vi "ADC SNR_Sweep_edited.vi"(8 "error in (no error)":errorcluster, 9 "Sequence parameters":string[][](array[string])=[["Min limit", "Max limit", "Register sheet file", "Register Sheet"], ["", "", "CC2600.xls", "TX_BLE;Trim"], ["Reg write (addr;value)", "Operating frequency [Hz]", "", ""], ["NA", "2.44G", "", ""]], 10 "Run type":i32, 11 "Method parameters":T3={"Dev"={"Do not disturb DUT"=FALSE, "XOSC"=32000000.0, "Board type"="", "EM"="", "Configure tempboard"=TRUE, "Device specific info"=[], "Generic Object"=refnum}, "Method"={"Run type"=1, "Test name"="Current LPM2 4", "Comment"="", "Results folder"="", "AFC"=enum."Off", "Method name"="Current LPM2 4", "Method results"={"Excel brief report"=FALSE, "Spotfire report"=FALSE, "Starfish report"=FALSE}, "Operator"="", "Reference time"=timestamp(0 s since 1904-01-01), "AFC delay"=0.0, "Initialization"=enum."Enabled", "MD5 Sum"="", "HW addon board"=enum."None", "AFC Regsheet"="", "AFC Regfile"=path "", "dummy"=0.0}, "Inst"={"Instr"={"PS1"={"Name"="", "GPIB address"="", "VISA session"=""}, "PS2"={"Name"="", "GPIB address"="", "VISA session"=""}, "TC1"={"Name"="", "GPIB address"="", "VISA session"=""}, "TC2"={"Name"="", "GPIB address"="", "VISA session"=""}, "SA1"={"Name"="", "GPIB address"="", "VISA session"=""}, "SA2"={"Name"="", "GPIB address"="", "VISA session"=""}, "SG1"={"Name"="", "GPIB address"="", "VISA session"=""}, "SG2"={"Name"="", "GPIB address"="", "VISA session"=""}, "SG3"={"Name"="", "GPIB address"="", "VISA session"=""}, "MI1"={"Name"="", "GPIB address"="", "VISA session"=""}, "MI2"={"Name"="", "GPIB address"="", "VISA session"=""}, "SW SA"={"Name"="", "Controller addr"=""}, "SW SG"={"Name"="", "Controller addr"=""}, "MI3"={"Name"="", "GPIB address"="", "VISA session"=""}}, "Switchbox"={"RF Path"=0, "Cal compensation"=enum."TX", "Switchbox gain mode"="", "State"=enum."TX"}, "Instr to control (i.e. SA1)"="Default", "Intrument info string"=""}, "Sequence parameters"=[["Weight", "Min Limit", "Max Limit", "Register Sheet", "", "", "", "", "", "", "", "", ""], ["Vital", "", "1", "LPM2", "", "", "", "", "", "", "", "", ""], ["Resolution", "Reg write (addr;value)", "Chip mode", "Range", "", "", "", "", "", "", "", "", ""], ["u", "NA", "", "auto", "", "", "", "", "", "", "", "", ""]], "Cond"={"Temp logged"=25.0, "VDD1_PS1_6V"=-999.0, "VDD2_PS1_25V"=-999.0, "VDD4_PS2_25V"=-999.0, "VDD3_PS2_6V"=-999.0}, "Meas config"={"X-axis inner loop index"=32000000, "Y-axis outer loop index"=32000000, "X-axis"=[], "Y-axis"=[], "X-axis array req size"=32000000, "Y-axis array req size"=32000000, "Param description"=[], "Use meas clust for reporting"=FALSE, "Parameter index (page)"=0, "X-axis name"="", "Y-axis name"=""}} {"Cond"."VDD3_PS2_6V" format="%.3f"; "Cond"."VDD4_PS2_25V" format="%.3f"; "Cond"."VDD2_PS1_25V" format="%.3f"; "Cond"."VDD1_PS1_6V" format="%.3f"; "Method"."dummy" format="%.1p"; "Method"."AFC delay" format="%.1p"; "Dev"."XOSC" format="%.3p"}) -> (0 "error out":errorcluster, 1 "End method error":T1, 2 "Short Results":string[](array[string]), 3 "Result summary":string[][](array[string])=[["Critical", "Output Power@2405 MHz", "-3", "4", "dBm"], ["Critical", "Output Power@2410 MHz", "-3", "4", "dBm"]])   [LabVIEW 2019]
doc: "[AutoDocStart]Performs crystal accuracy measurements. Measures the offset from ideal frequency. Primarily used for tuning XOSC capacitors and verifying XOSC trims.\n\nSweeping parameters: operating frequency, OSC override value and VDDR level\n\nResults: Offset frequency in ppm[AutoDocEnd]"
uses:
  User Lib/Utilities/Cluster definitions/Method input.ctl
  User Lib/Utilities/Cluster definitions/Device specific info.ctl
  User Lib/Utilities/Controls/Automatic Frequency Compensation types.ctl
  User Lib/Utilities/Controls/Method Reports.ctl
  User Lib/Utilities/Cluster definitions/Method Initialization.ctl
  User Lib/Utilities/Controls/HW addon boards.ctl
  User Lib/Utilities/Cluster definitions/Instr clust.ctl
  User Lib/Utilities/Switchbox control/SwitchBox_State._ENUMctl.ctl
  User Lib/Utilities/Cluster definitions/End method error cluster.ctl
  d1e189ac-5c6c-49e1-a56b-a93f7ba1e5c3.vi
  89ac9e08-f822-48c3-bf7b-b9620a48f2c1.vi
  afbe0b8a-4628-4f4a-a689-fb3560c1b1a6.vi
  160c279e-5860-4c4e-a522-43dd8a66307b.vi
  eb3a7dab-0138-448e-bc0a-4bb49588a4f1.vi
  4ae92598-944e-459b-8fa7-3a23a971f601.vi
  e1f832d6-75bf-4ba2-931c-48c142ce58ac.vi
panel:
  in  "Tab Control":T2(tab)
  # "°C"
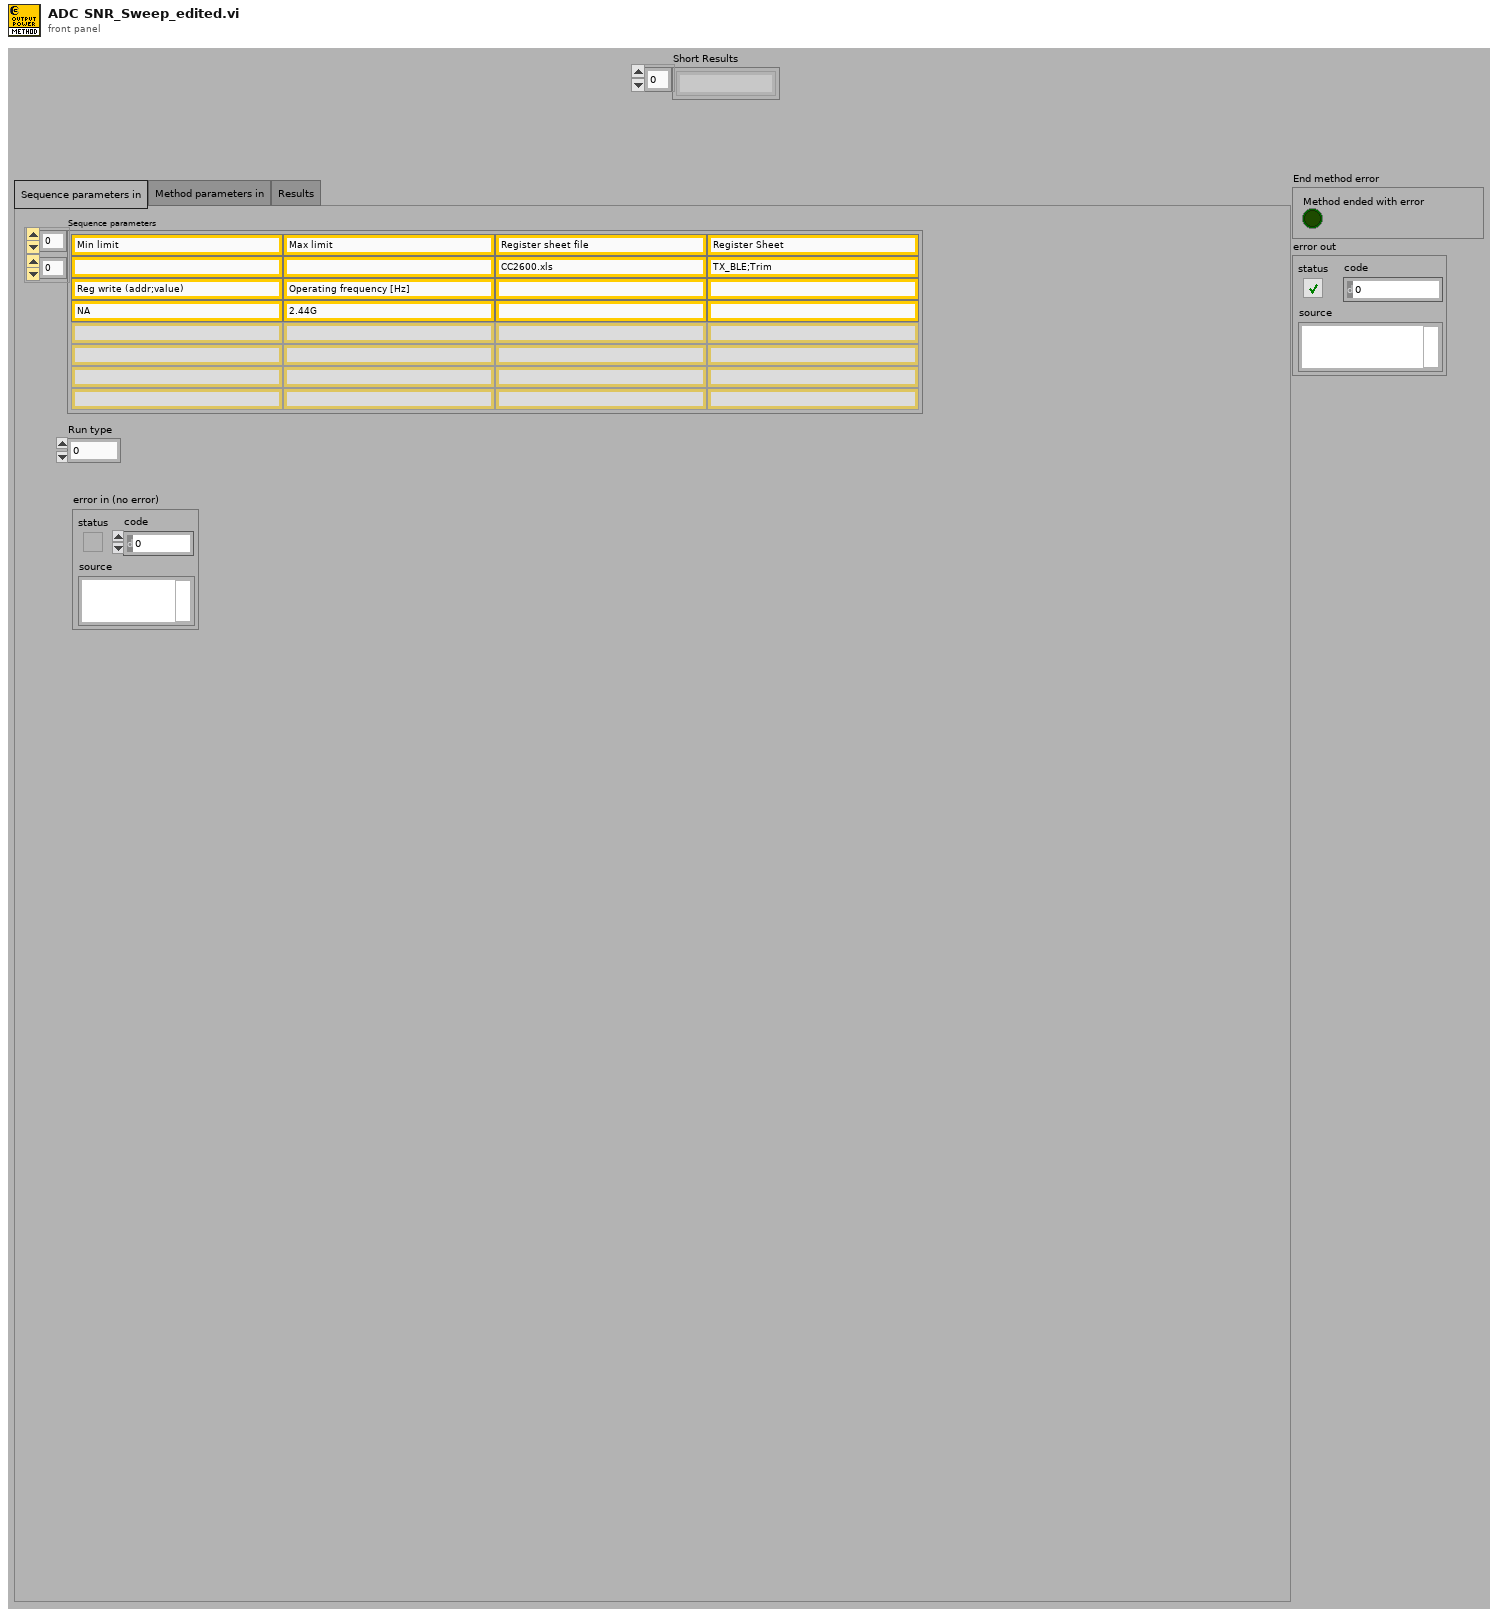
[diagram p1: front panel]
types:
  T1 = typedef "End method error cluster.ctl" = cluster{"Method ended with error":bool}
  T2 = enum32{"Sequence parameters in", "Method parameters in", "Results"}
  T3 = typedef "Method input.ctl" = cluster{"Dev":cluster{"Do not disturb DUT":bool, "XOSC":dbl, "Board type":string, "EM":string, "Configure tempboard":bool, "Device specific info":T4[], "Generic Object":refnum<class>}, "Method":cluster{"Run type":i32, "Test name":string, "Comment":string, "Results folder":string, "AFC":T5, "Method name":string, "Method results":T6, "Operator":string, "Reference time":timestamp, "AFC delay":dbl, "Initialization":T7, "MD5 Sum":string, "HW addon board":T8, "AFC Regsheet":string, "AFC Regfile":path, "dummy":dbl}, "Inst":T9, "Sequence parameters":string[][], "Cond":cluster{"Temp logged":dbl, "VDD1_PS1_6V":dbl, "VDD2_PS1_25V":dbl, "VDD4_PS2_25V":dbl, "VDD3_PS2_6V":dbl}, "Meas config":cluster{"X-axis inner loop index":i32, "Y-axis outer loop index":i32, "X-axis":string[], "Y-axis":string[], "X-axis array req size":i32, "Y-axis array req size":i32, "Param description":string[][], "Use meas clust for reporting":bool, "Parameter index (page)":i32, "X-axis name":string, "Y-axis name":string}}
  T4 = typedef "Device specific info.ctl" = cluster{"EM number":u8, "IP address":string, "Enabled":bool, "Slot no":u8, "RF path":u8, "EM name":string, "Wafer info":string, "AFC frequency ppm":dbl, "Register writes":string[][], "Meas data":string[][][], "Device comment":string}
  T5 = typedef "Automatic Frequency Compensation types.ctl" = enum16{"Off", "Compensate Instrument frequency", "Compensate DUT frequency", "Predictive - Compensate Instrument frequency", "Predictive - Compensate DUT frequency", "Do not skip re-init - Compensate Instrument frequency", "Do not skip re-init - Compensate DUT frequency"}
  T6 = typedef "Method Reports.ctl" = cluster{"Excel brief report":bool, "Spotfire report":bool, "Starfish report":bool}
  T7 = typedef "Method Initialization.ctl" = enum16{"Enabled", "Skip Instr and Device Init", "Enabled with Separate Flash", "Set PS, Device Init and Skip Instr Init", "Skip Device Init"}
  T8 = typedef "HW addon boards.ctl" = enum16{"None", "Current meas 5EM", "Stresstest 10EM"}
  T9 = typedef "Instr clust.ctl" = cluster{"Instr":cluster{"PS1":cluster{"Name":string, "GPIB address":string, "VISA session":refnum<visa-resource-name>}, "PS2":cluster{"Name":string, "GPIB address":string, "VISA session":refnum<visa-resource-name>}, "TC1":cluster{"Name":string, "GPIB address":string, "VISA session":refnum<visa-resource-name>}, "TC2":cluster{"Name":string, "GPIB address":string, "VISA session":refnum<visa-resource-name>}, "SA1":cluster{"Name":string, "GPIB address":string, "VISA session":refnum<visa-resource-name>}, "SA2":cluster{"Name":string, "GPIB address":string, "VISA session":refnum<visa-resource-name>}, "SG1":cluster{"Name":string, "GPIB address":string, "VISA session":refnum<visa-resource-name>}, "SG2":cluster{"Name":string, "GPIB address":string, "VISA session":refnum<visa-resource-name>}, "SG3":cluster{"Name":string, "GPIB address":string, "VISA session":refnum<visa-resource-name>}, "MI1":cluster{"Name":string, "GPIB address":string, "VISA session":refnum<visa-resource-name>}, "MI2":cluster{"Name":string, "GPIB address":string, "VISA session":refnum<visa-resource-name>}, "SW SA":cluster{"Name":string, "Controller addr":string}, "SW SG":cluster{"Name":string, "Controller addr":string}, "MI3":cluster{"Name":string, "GPIB address":string, "VISA session":refnum<visa-resource-name>}}, "Switchbox":cluster{"RF Path":i32, "Cal compensation":enum16{"TX", "RX", "Interferer", "No compensation", "Interferer2"}, "Switchbox gain mode":string, "State":T10}, "Instr to control (i.e. SA1)":string, "Intrument info string":string}
  T10 = typedef "SwitchBox_State._ENUMctl.ctl" = enum16{"TX", "RX", "SP:TX", "SP:RX", "SW:TX", "SW:RX"}
  T11 = cluster{"Fundamental Frequency":dbl, "Sampling Frequncy":dbl, "No of Harmonics":u8, "Window":enum16{"None ", "Hanning", "Hamming", "Blackman-Harris", "Exact Blackman", "Blackman", "Flat Top", "4 Term B-Harris ", "7 Term B-Harris"}, "Blackman (fundamental power) bins)":dbl}
  T12 = enum32{"NI Card Settings", "Memory Read Setting", "DC Capture", "ADC Ramp", "ADC Sine", "SNR", "Cap Calibration"}
  T13 = enum32{"Read from Memory", "Read .dat file", "NI Card Capture", "None"}
  T14 = cluster{"Path to Save plot":path, "Path to Raw Data plot":path}
  T15 = cluster{"Save INL/DNL Plot(Ramp)":bool, "Save SNR Plot":bool, "Save INL/DNL Plot(Sine)":bool, "Save INL/DNL Raw Data(Ramp)":bool, "Save SNR Raw Data":bool, "Save INL/DNL Raw Data(Sine)":bool, "Save DC Raw data":bool, "Save  Raw Data(Sine)":bool}
  T16 = cluster{"SNR":dbl, "SNRD":dbl, "THD":dbl, "ENOB (SNRD)":dbl, "SFDR":dbl, "ENOB (SNR)":dbl, "Noise Power":dbl, "Signal power":dbl}
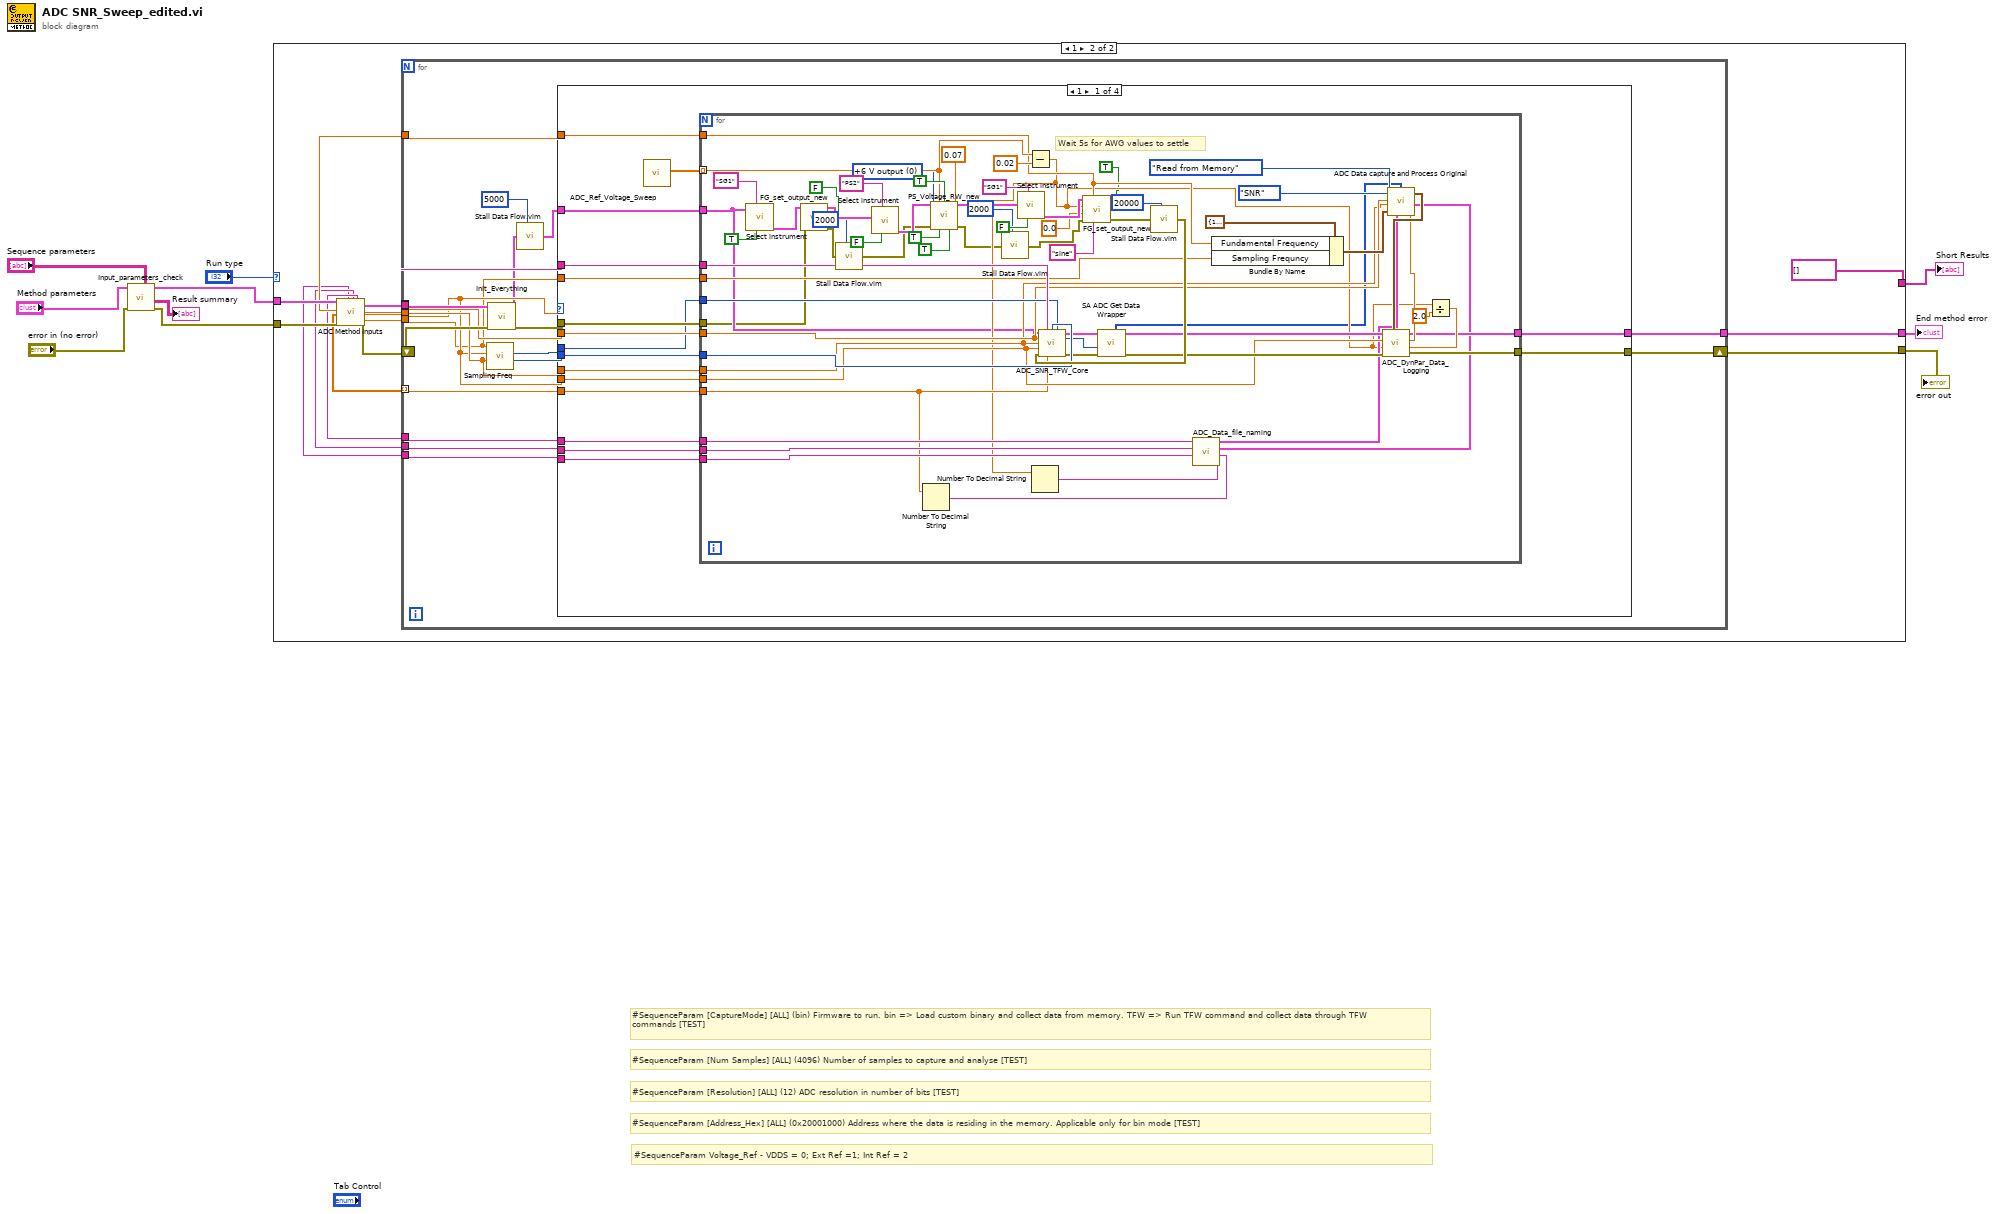
[diagram p0: block diagram]
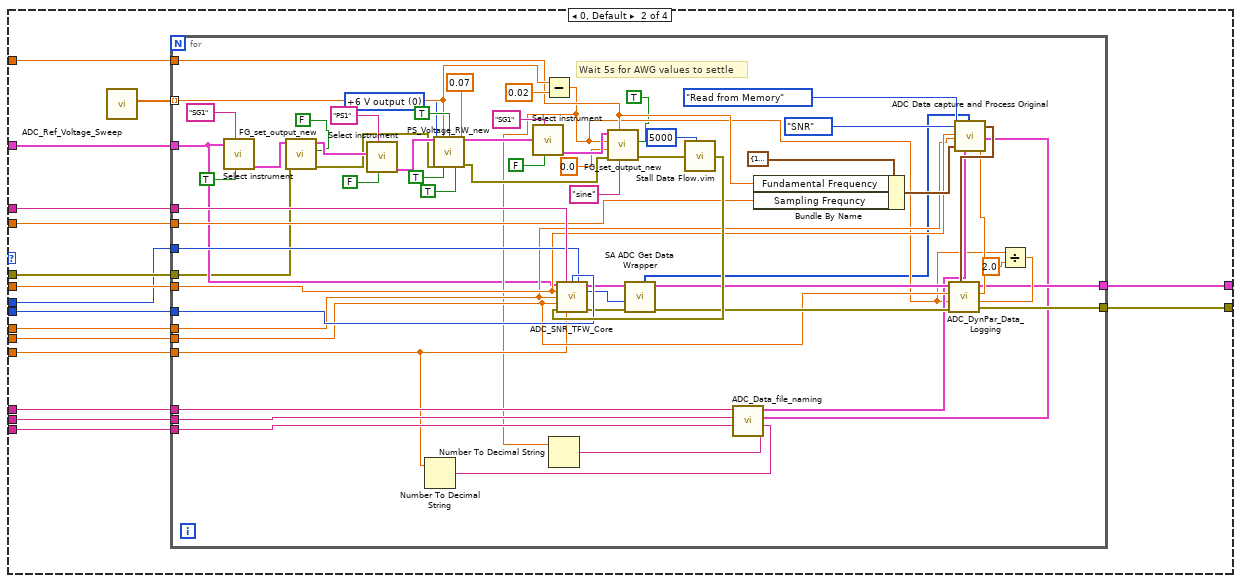
[diagram p3: hidden frame]
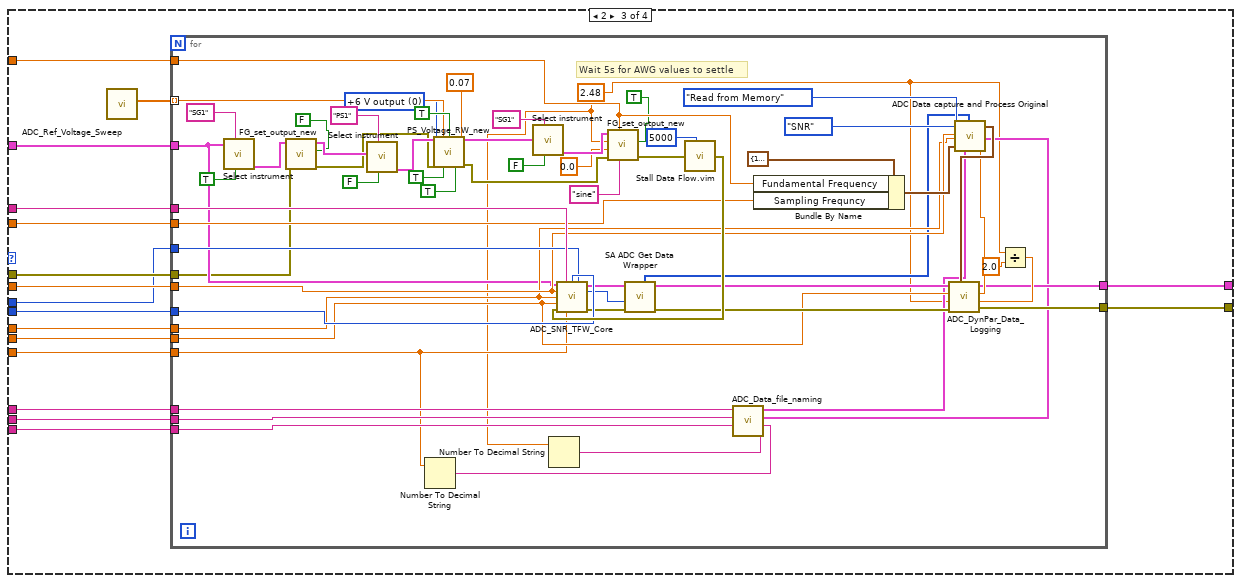
[diagram p4: hidden frame]
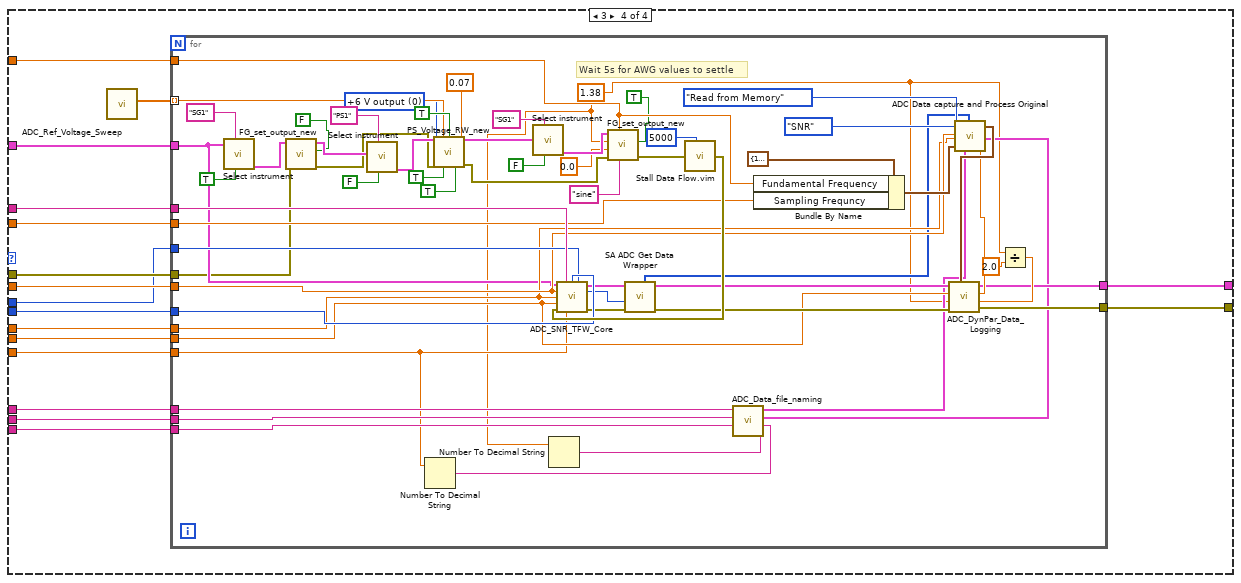
[diagram p5: hidden frame]
diagram:
  # "#SequenceParam Voltage_Ref - VDDS = 0; Ext Ref =1; Int Ref = 2"
  # "#SequenceParam [Num Samples] [ALL] (4096) Number of samples to capture and analyse [TEST]"
  # "#SequenceParam [CaptureMode] [ALL] (bin) Firmware to run. bin => Load custom binary and collect data from memory. TFW => Run TFW command and collect data through TFW commands [TEST]"
  # "#SequenceParam [Address_Hex] [ALL] (0x20001000) Address where the data is residing in the memory. Applicable only for bin mode [TEST]"
  # "#SequenceParam [Resolution] [ALL] (12) ADC resolution in number of bits [TEST]"
  n1 = call "Input_parameters_check.vi"("Sequence parameters"="Sequence parameters", "error in"="error in (no error)", "Method cluster in"="Method parameters") -> ("error out"=w10:errorcluster, "Result summary"=→"Result summary":string[][], "Method cluster out"=w6:T3)  [unwired: 6 in]
  n2 = case shown="1" "Run type" {
    tunnel: w10 -> [w11 w28]
    tunnel: w6 -> [_ w27]
    tunnel: [string[] [] string[] []] -> w3
    tunnel: [w11 w18] -> w2
    tunnel: [_ w17] -> w1
    frame 0, Default {
      # "Run type 0 is only for formatting the result summary"
    }
    frame 1 {
      n3 = call "ADC Method Inputs.vi"("Method cluster in"=w27, "error in (no error)"=w28) -> ("Capture Mode"=w21:string, "Signal Freq"=w20:dbl, "ADC Chnl No."=w13:dbl[], "Sampling Freq String"=w14:string, "Resolution String"=w15:string, "Voltage Ref String"=w16:string, "Method cluster out"=w26:T3, "Num Samples"=w24:dbl, "Resolution"=w23:dbl, "Voltage Ref"=w22:dbl, "Sampling Freq"=w19:dbl, "error out"=w25:errorcluster)  [unwired: 6 in]
      n4 = for {
        tunnel: w26 -> [w49]
        tunnel: w24 -> [w46]
        tunnel: w23 -> [w45]
        tunnel: w22 -> [w44]
        tunnel: w21 -> [w43]
        tunnel: w20 -> [w40]
        tunnel: w19 -> [w39]
        tunnel: [w37] -> w17
        tunnel: w16 -> [w36]
        tunnel: w15 -> [w35]
        tunnel: w14 -> [w34]
        shift-right: [w38] -> w18
        shift-left: w25 -> [w48]
        tunnel: w13 -> [w33] mode=indexing
        n5 = call "Sampling Freq.vi"("Resolution"=w45, "Voltage Ref"=w44, "Sampling Freq"=w39) -> ("LGPT Count"=w42:u16, "SCOMP"=w41:u16)  [unwired: 7 in]
        n6 = call "Init_Everything.vi"("error in"=w48, "Method cluster In"=w49) -> ("error out"=w47:errorcluster, "Method cluster out"=w31:T3)  [unwired: 6 in, 2 out]
        n7 = call "Stall Data Flow.vim"("value in"=w31, "milliseconds to wait"=u32 5000) -> ("value out"=w32:T3)  [unwired: 1 out]
        n8 = case shown="1" w44 {
          tunnel: w32 -> [w65 w148 w227 w305]
          tunnel: w47 -> [w64 w147 w226 w304]
          tunnel: w46 -> [w63 w146 w225 w303]
          tunnel: w45 -> [w62 w145 w224 w302]
          tunnel: w44 -> [w61 w144 w223 w301]
          tunnel: w43 -> [w60 w143 w222 w300]
          tunnel: w42 -> [w59 w142 w221 w299]
          tunnel: w41 -> [w58 w141 w220 w298]
          tunnel: w40 -> [w57 w140 w219 w297]
          tunnel: w33 -> [w56 w139 w218 w296]
          tunnel: w39 -> [w55 w138 w217 w295]
          tunnel: [w54 w137 w216 w294] -> w37
          tunnel: [w53 w136 w215 w293] -> w38
          tunnel: w36 -> [w52 w135 w214 w292]
          tunnel: w35 -> [w51 w134 w213 w291]
          tunnel: w34 -> [w50 w133 w212 w290]
          frame 1 {
            n9 = call "ADC_Ref_Voltage_Sweep.vi"() -> ("Ref voltage sweep"=w66:dbl[])  [unwired: 11 in]
            n10 = for {
              tunnel: w66 -> [w112] mode=indexing
              tunnel: w65 -> [w81]
              tunnel: w64 -> [w77]
              tunnel: w63 -> [w102]
              tunnel: w62 -> [w101]
              tunnel: w61 -> [w96]
              tunnel: w60 -> [w115]
              tunnel: w59 -> [w114]
              tunnel: w58 -> [w113]
              tunnel: w57 -> [w105]
              tunnel: w56 -> [w86]
              tunnel: w55 -> [w104]
              tunnel: [w93] -> w54
              tunnel: [w92] -> w53
              tunnel: w52 -> [w89]
              tunnel: w51 -> [w88]
              tunnel: w50 -> [w87]
              w73 = u16 0 items=["+6 V output", "+25 V output", "-25 V output", "ALL TERM"] ("Output Terminals")
              # "Wait 5s for AWG values to settle"
              n11 = call "Select instrument.vi"("Method cluster (T) / Instr cluster (F)"=TRUE, "Instr.Instr to control (i.e. SA1)"="SG1", "Method cluster in"=w81) -> ("Instr out"=w80:T9)  [unwired: 6 in, 2 out]
              n12 = call "FG_set_output_new.vi"("Enable Output?"=FALSE, "error in"=w77, "InstrCluster in"=w80) -> ("error out"=w72:errorcluster, "InstrCluster out"=w78:T9)  [unwired: 7 in]
              n13 = call "Stall Data Flow.vim"("value in"=w72, "milliseconds to wait"=u32 2000) -> ("value out"=w71:errorcluster)  [unwired: 1 out]
              n14 = call "Select instrument.vi"("Method cluster (T) / Instr cluster (F)"=FALSE, "Instr.Instr to control (i.e. SA1)"="PS2", "Instr in"=w78) -> ("Instr out"=w123:T9)  [unwired: 6 in, 2 out]
              n15 = Number To Decimal String(number=w86) -> (decimal integer string=w85:string)  [unwired: 1 in]
              n16 = call "PS_Voltage_RW_new.vi"("InstrCluster in"=w123, "Set Voltage"=w112, "Limit to 4V (T)"=TRUE, "Current(0)"=0.07, "Output Terminals"=w73, "error in (no error)"=w71, "Off (F)                         On (T)"=TRUE, "Read (F)                      Write (T)"=TRUE) -> ("InstrCluster out"=w124:T9, "error out"=w69:errorcluster)  [unwired: 5 in, 1 out]
              n17 = call "Stall Data Flow.vim"("value in"=w69, "milliseconds to wait"=u32 2000) -> ("value out"=w68:errorcluster)  [unwired: 1 out]
              n18 = call "Select instrument.vi"("Method cluster (T) / Instr cluster (F)"=FALSE, "Instr.Instr to control (i.e. SA1)"="SG1", "Instr in"=w124) -> ("Instr out"=w127:T9)  [unwired: 6 in, 2 out]
              n19 = Subtract(x=w112, y=0.02) -> (x-y=w84:dbl)
              n20 = Number To Decimal String(number=w84) -> (decimal integer string=w83:string)  [unwired: 1 in]
              n21 = call "FG_set_output_new.vi"("Enable Output?"=TRUE, "Function (DC, Sine, Square, Triangle, Ramp up, Ramp down, Pulse)"="sine", "Frequency [Hz]"=w105, "error in"=w68, "Low voltage"=0.0, "High voltage (or DC)"=w84, "InstrCluster in"=w127) -> ("error out"=w117:errorcluster)  [unwired: 3 in, 1 out]
              n22 = call "Stall Data Flow.vim"("value in"=w117, "milliseconds to wait"=u32 20000) -> ("value out"=w116:errorcluster)  [unwired: 1 out]
              n23 = call "ADC_SNR_TFW_Core.vi"("Method cluster in"=w81, "Capture Mode"=w115, "LGPT Count"=w114, "SCOMP"=w113, "No. Samples"=w102, "Resolution"=w101, "Voltage Ref"=w96, "error in"=w116, "ADC Chnl No."=w86) -> ("Method cluster out 2"=w110:T3, "ResPar[0] Data Address"=w109:u32, "error out"=w111:errorcluster)  [unwired: 3 in, 1 out]
              n24 = call "SA ADC Get Data Wrapper.vi"("error in"=w111, "Data Address"=w109, "Method cluster in"=w110) -> ("error out"=w98:errorcluster, "output cluster"=w99:T3, "ADC samples"=w82:u32[])  [unwired: 3 in, 3 out]
              n25 = call "ADC_Data_file_naming.vi"("Amplitude (Vpp)"=w83, "ADC Chn. No"=w85, "Sampling Freq String"=w87, "Resolution String"=w88, "Voltage Ref String"=w89) -> ("path to save"=w90:T14, "Save data"=w91:T15)  [unwired: 5 in]
              n26 = Bundle By Name(cluster=T11 {"Fundamental Frequency"=10000.0, "Sampling Frequncy"=250000.0, "No of Harmonics"=9, "Window"=enum."7 Term B-Harris", "Blackman (fundamental power) bins)"=1.0} ("Inputs for Dyanmic para"), "Fundamental Frequency"=w105, "Sampling Frequncy"=w104) -> (w103:T11)
              n27 = call "ADC Data capture and Process Original.vi"("ADC Output Read Method"=T13."Read from Memory", "Select the Tab to project"=T12."SNR", "No.of samples(SNR)"=w102, "Resolution"=w101, "Inputs for Dyanmic para"=w103, "Save data"=w91, "Waveform"=w82, "path to save"=w90) -> ("detected Throughput"=w97:dbl, "Dynamic Parameters"=w100:T16)  [unwired: 13 in, 5 out]
              n28 = Divide(x=w84, y=2.0) -> (x/y=w94:dbl)
              n29 = call "ADC_DynPar_Data_Logging.vi"("Offset (V)"=w94, "detected Throughput"=w97, "Dynamic Parameters"=w100, "error in (no error)"=w98, "Amplitude (Vpp)"=w84, "Ref Voltage"=w96, "Method Cluster In"=w99) -> ("error out"=w92:errorcluster, "End method error"=w93:T1)  [unwired: 3 in]
            }
          }
          frame 0, Default {
            n30 = call "ADC_Ref_Voltage_Sweep.vi"() -> ("Ref voltage sweep"=w149:dbl[])  [unwired: 11 in]
            n31 = for {
              tunnel: w149 -> [w190] mode=indexing
              tunnel: w148 -> [w159]
              tunnel: w147 -> [w155]
              tunnel: w146 -> [w180]
              tunnel: w145 -> [w179]
              tunnel: w144 -> [w174]
              tunnel: w143 -> [w193]
              tunnel: w142 -> [w192]
              tunnel: w141 -> [w191]
              tunnel: w140 -> [w183]
              tunnel: w139 -> [w164]
              tunnel: w138 -> [w182]
              tunnel: [w171] -> w137
              tunnel: [w170] -> w136
              tunnel: w135 -> [w167]
              tunnel: w134 -> [w166]
              tunnel: w133 -> [w165]
              w150 = u16 0 items=["+6 V output", "+25 V output", "-25 V output", "ALL TERM"] ("Output Terminals")
              # "Wait 5s for AWG values to settle"
              n32 = call "Select instrument.vi"("Method cluster (T) / Instr cluster (F)"=TRUE, "Instr.Instr to control (i.e. SA1)"="SG1", "Method cluster in"=w159) -> ("Instr out"=w158:T9)  [unwired: 6 in, 2 out]
              n33 = call "FG_set_output_new.vi"("Enable Output?"=FALSE, "error in"=w155, "InstrCluster in"=w158) -> ("error out"=w154:errorcluster, "InstrCluster out"=w156:T9)  [unwired: 7 in]
              n34 = call "Select instrument.vi"("Method cluster (T) / Instr cluster (F)"=FALSE, "Instr.Instr to control (i.e. SA1)"="PS1", "Instr in"=w156) -> ("Instr out"=w201:T9)  [unwired: 6 in, 2 out]
              n35 = Number To Decimal String(number=w164) -> (decimal integer string=w163:string)  [unwired: 1 in]
              n36 = call "PS_Voltage_RW_new.vi"("InstrCluster in"=w201, "Set Voltage"=w190, "Limit to 4V (T)"=TRUE, "Current(0)"=0.07, "Output Terminals"=w150, "error in (no error)"=w154, "Off (F)                         On (T)"=TRUE, "Read (F)                      Write (T)"=TRUE) -> ("InstrCluster out"=w202:T9, "error out"=w203:errorcluster)  [unwired: 5 in, 1 out]
              n37 = call "Select instrument.vi"("Method cluster (T) / Instr cluster (F)"=FALSE, "Instr.Instr to control (i.e. SA1)"="SG1", "Instr in"=w202) -> ("Instr out"=w206:T9)  [unwired: 6 in, 2 out]
              n38 = Subtract(x=w190, y=0.02) -> (x-y=w162:dbl)
              n39 = Number To Decimal String(number=w162) -> (decimal integer string=w161:string)  [unwired: 1 in]
              n40 = call "FG_set_output_new.vi"("Enable Output?"=TRUE, "Function (DC, Sine, Square, Triangle, Ramp up, Ramp down, Pulse)"="sine", "Frequency [Hz]"=w183, "error in"=w203, "Low voltage"=0.0, "High voltage (or DC)"=w162, "InstrCluster in"=w206) -> ("error out"=w195:errorcluster)  [unwired: 3 in, 1 out]
              n41 = call "Stall Data Flow.vim"("value in"=w195, "milliseconds to wait"=u32 5000) -> ("value out"=w194:errorcluster)  [unwired: 1 out]
              n42 = call "ADC_SNR_TFW_Core.vi"("Method cluster in"=w159, "Capture Mode"=w193, "LGPT Count"=w192, "SCOMP"=w191, "No. Samples"=w180, "Resolution"=w179, "Voltage Ref"=w174, "error in"=w194, "ADC Chnl No."=w164) -> ("Method cluster out 2"=w188:T3, "ResPar[0] Data Address"=w187:u32, "error out"=w189:errorcluster)  [unwired: 3 in, 1 out]
              n43 = call "SA ADC Get Data Wrapper.vi"("error in"=w189, "Data Address"=w187, "Method cluster in"=w188) -> ("error out"=w176:errorcluster, "output cluster"=w177:T3, "ADC samples"=w160:u32[])  [unwired: 3 in, 3 out]
              n44 = call "ADC_Data_file_naming.vi"("Amplitude (Vpp)"=w161, "ADC Chn. No"=w163, "Sampling Freq String"=w165, "Resolution String"=w166, "Voltage Ref String"=w167) -> ("path to save"=w168:T14, "Save data"=w169:T15)  [unwired: 5 in]
              n45 = Bundle By Name(cluster=T11 {"Fundamental Frequency"=10000.0, "Sampling Frequncy"=250000.0, "No of Harmonics"=9, "Window"=enum."7 Term B-Harris", "Blackman (fundamental power) bins)"=1.0} ("Inputs for Dyanmic para"), "Fundamental Frequency"=w183, "Sampling Frequncy"=w182) -> (w181:T11)
              n46 = call "ADC Data capture and Process Original.vi"("ADC Output Read Method"=T13."Read from Memory", "Select the Tab to project"=T12."SNR", "No.of samples(SNR)"=w180, "Resolution"=w179, "Inputs for Dyanmic para"=w181, "Save data"=w169, "Waveform"=w160, "path to save"=w168) -> ("detected Throughput"=w175:dbl, "Dynamic Parameters"=w178:T16)  [unwired: 13 in, 5 out]
              n47 = Divide(x=w162, y=2.0) -> (x/y=w172:dbl)
              n48 = call "ADC_DynPar_Data_Logging.vi"("Offset (V)"=w172, "detected Throughput"=w175, "Dynamic Parameters"=w178, "error in (no error)"=w176, "Amplitude (Vpp)"=w162, "Ref Voltage"=w174, "Method Cluster In"=w177) -> ("error out"=w170:errorcluster, "End method error"=w171:T1)  [unwired: 3 in]
            }
          }
          frame 2 {
            n49 = call "ADC_Ref_Voltage_Sweep.vi"() -> ("Ref voltage sweep"=w228:dbl[])  [unwired: 11 in]
            n50 = for {
              tunnel: w228 -> [w269] mode=indexing
              tunnel: w227 -> [w239]
              tunnel: w226 -> [w235]
              tunnel: w225 -> [w259]
              tunnel: w224 -> [w258]
              tunnel: w223 -> [w253]
              tunnel: w222 -> [w272]
              tunnel: w221 -> [w271]
              tunnel: w220 -> [w270]
              tunnel: w219 -> [w262]
              tunnel: w218 -> [w243]
              tunnel: w217 -> [w261]
              tunnel: [w250] -> w216
              tunnel: [w249] -> w215
              tunnel: w214 -> [w246]
              tunnel: w213 -> [w245]
              tunnel: w212 -> [w244]
              w229 = u16 0 items=["+6 V output", "+25 V output", "-25 V output", "ALL TERM"] ("Output Terminals")
              w230 = 2.48
              # "Wait 5s for AWG values to settle"
              n51 = call "Select instrument.vi"("Method cluster (T) / Instr cluster (F)"=TRUE, "Instr.Instr to control (i.e. SA1)"="SG1", "Method cluster in"=w239) -> ("Instr out"=w238:T9)  [unwired: 6 in, 2 out]
              n52 = call "FG_set_output_new.vi"("Enable Output?"=FALSE, "error in"=w235, "InstrCluster in"=w238) -> ("error out"=w234:errorcluster, "InstrCluster out"=w236:T9)  [unwired: 7 in]
              n53 = call "Select instrument.vi"("Method cluster (T) / Instr cluster (F)"=FALSE, "Instr.Instr to control (i.e. SA1)"="PS1", "Instr in"=w236) -> ("Instr out"=w280:T9)  [unwired: 6 in, 2 out]
              n54 = Number To Decimal String(number=w243) -> (decimal integer string=w242:string)  [unwired: 1 in]
              n55 = call "PS_Voltage_RW_new.vi"("InstrCluster in"=w280, "Set Voltage"=w269, "Limit to 4V (T)"=TRUE, "Current(0)"=0.07, "Output Terminals"=w229, "error in (no error)"=w234, "Off (F)                         On (T)"=TRUE, "Read (F)                      Write (T)"=TRUE) -> ("InstrCluster out"=w281:T9, "error out"=w282:errorcluster)  [unwired: 5 in, 1 out]
              n56 = call "Select instrument.vi"("Method cluster (T) / Instr cluster (F)"=FALSE, "Instr.Instr to control (i.e. SA1)"="SG1", "Instr in"=w281) -> ("Instr out"=w285:T9)  [unwired: 6 in, 2 out]
              n57 = Number To Decimal String(number=w230) -> (decimal integer string=w241:string)  [unwired: 1 in]
              n58 = call "FG_set_output_new.vi"("Enable Output?"=TRUE, "Function (DC, Sine, Square, Triangle, Ramp up, Ramp down, Pulse)"="sine", "Frequency [Hz]"=w262, "error in"=w282, "Low voltage"=0.0, "High voltage (or DC)"=w230, "InstrCluster in"=w285) -> ("error out"=w274:errorcluster)  [unwired: 3 in, 1 out]
              n59 = call "Stall Data Flow.vim"("value in"=w274, "milliseconds to wait"=u32 5000) -> ("value out"=w273:errorcluster)  [unwired: 1 out]
              n60 = call "ADC_SNR_TFW_Core.vi"("Method cluster in"=w239, "Capture Mode"=w272, "LGPT Count"=w271, "SCOMP"=w270, "No. Samples"=w259, "Resolution"=w258, "Voltage Ref"=w253, "error in"=w273, "ADC Chnl No."=w243) -> ("Method cluster out 2"=w267:T3, "ResPar[0] Data Address"=w266:u32, "error out"=w268:errorcluster)  [unwired: 3 in, 1 out]
              n61 = call "SA ADC Get Data Wrapper.vi"("error in"=w268, "Data Address"=w266, "Method cluster in"=w267) -> ("error out"=w255:errorcluster, "output cluster"=w256:T3, "ADC samples"=w240:u32[])  [unwired: 3 in, 3 out]
              n62 = call "ADC_Data_file_naming.vi"("Amplitude (Vpp)"=w241, "ADC Chn. No"=w242, "Sampling Freq String"=w244, "Resolution String"=w245, "Voltage Ref String"=w246) -> ("path to save"=w247:T14, "Save data"=w248:T15)  [unwired: 5 in]
              n63 = Bundle By Name(cluster=T11 {"Fundamental Frequency"=10000.0, "Sampling Frequncy"=250000.0, "No of Harmonics"=9, "Window"=enum."7 Term B-Harris", "Blackman (fundamental power) bins)"=1.0} ("Inputs for Dyanmic para"), "Fundamental Frequency"=w262, "Sampling Frequncy"=w261) -> (w260:T11)
              n64 = call "ADC Data capture and Process Original.vi"("ADC Output Read Method"=T13."Read from Memory", "Select the Tab to project"=T12."SNR", "No.of samples(SNR)"=w259, "Resolution"=w258, "Inputs for Dyanmic para"=w260, "Save data"=w248, "Waveform"=w240, "path to save"=w247) -> ("detected Throughput"=w254:dbl, "Dynamic Parameters"=w257:T16)  [unwired: 13 in, 5 out]
              n65 = Divide(x=w230, y=2.0) -> (x/y=w251:dbl)
              n66 = call "ADC_DynPar_Data_Logging.vi"("Offset (V)"=w251, "detected Throughput"=w254, "Dynamic Parameters"=w257, "error in (no error)"=w255, "Amplitude (Vpp)"=w230, "Ref Voltage"=w253, "Method Cluster In"=w256) -> ("error out"=w249:errorcluster, "End method error"=w250:T1)  [unwired: 3 in]
            }
          }
          frame 3 {
            n67 = call "ADC_Ref_Voltage_Sweep.vi"() -> ("Ref voltage sweep"=w306:dbl[])  [unwired: 11 in]
            n68 = for {
              tunnel: w306 -> [w347] mode=indexing
              tunnel: w305 -> [w317]
              tunnel: w304 -> [w313]
              tunnel: w303 -> [w337]
              tunnel: w302 -> [w336]
              tunnel: w301 -> [w331]
              tunnel: w300 -> [w350]
              tunnel: w299 -> [w349]
              tunnel: w298 -> [w348]
              tunnel: w297 -> [w340]
              tunnel: w296 -> [w321]
              tunnel: w295 -> [w339]
              tunnel: [w328] -> w294
              tunnel: [w327] -> w293
              tunnel: w292 -> [w324]
              tunnel: w291 -> [w323]
              tunnel: w290 -> [w322]
              w307 = u16 0 items=["+6 V output", "+25 V output", "-25 V output", "ALL TERM"] ("Output Terminals")
              w308 = 1.38
              # "Wait 5s for AWG values to settle"
              n69 = call "Select instrument.vi"("Method cluster (T) / Instr cluster (F)"=TRUE, "Instr.Instr to control (i.e. SA1)"="SG1", "Method cluster in"=w317) -> ("Instr out"=w316:T9)  [unwired: 6 in, 2 out]
              n70 = call "FG_set_output_new.vi"("Enable Output?"=FALSE, "error in"=w313, "InstrCluster in"=w316) -> ("error out"=w312:errorcluster, "InstrCluster out"=w314:T9)  [unwired: 7 in]
              n71 = call "Select instrument.vi"("Method cluster (T) / Instr cluster (F)"=FALSE, "Instr.Instr to control (i.e. SA1)"="PS1", "Instr in"=w314) -> ("Instr out"=w358:T9)  [unwired: 6 in, 2 out]
              n72 = Number To Decimal String(number=w321) -> (decimal integer string=w320:string)  [unwired: 1 in]
              n73 = call "PS_Voltage_RW_new.vi"("InstrCluster in"=w358, "Set Voltage"=w347, "Limit to 4V (T)"=TRUE, "Current(0)"=0.07, "Output Terminals"=w307, "error in (no error)"=w312, "Off (F)                         On (T)"=TRUE, "Read (F)                      Write (T)"=TRUE) -> ("InstrCluster out"=w359:T9, "error out"=w360:errorcluster)  [unwired: 5 in, 1 out]
              n74 = call "Select instrument.vi"("Method cluster (T) / Instr cluster (F)"=FALSE, "Instr.Instr to control (i.e. SA1)"="SG1", "Instr in"=w359) -> ("Instr out"=w363:T9)  [unwired: 6 in, 2 out]
              n75 = Number To Decimal String(number=w308) -> (decimal integer string=w319:string)  [unwired: 1 in]
              n76 = call "FG_set_output_new.vi"("Enable Output?"=TRUE, "Function (DC, Sine, Square, Triangle, Ramp up, Ramp down, Pulse)"="sine", "Frequency [Hz]"=w340, "error in"=w360, "Low voltage"=0.0, "High voltage (or DC)"=w308, "InstrCluster in"=w363) -> ("error out"=w352:errorcluster)  [unwired: 3 in, 1 out]
              n77 = call "Stall Data Flow.vim"("value in"=w352, "milliseconds to wait"=u32 5000) -> ("value out"=w351:errorcluster)  [unwired: 1 out]
              n78 = call "ADC_SNR_TFW_Core.vi"("Method cluster in"=w317, "Capture Mode"=w350, "LGPT Count"=w349, "SCOMP"=w348, "No. Samples"=w337, "Resolution"=w336, "Voltage Ref"=w331, "error in"=w351, "ADC Chnl No."=w321) -> ("Method cluster out 2"=w345:T3, "ResPar[0] Data Address"=w344:u32, "error out"=w346:errorcluster)  [unwired: 3 in, 1 out]
              n79 = call "SA ADC Get Data Wrapper.vi"("error in"=w346, "Data Address"=w344, "Method cluster in"=w345) -> ("error out"=w333:errorcluster, "output cluster"=w334:T3, "ADC samples"=w318:u32[])  [unwired: 3 in, 3 out]
              n80 = call "ADC_Data_file_naming.vi"("Amplitude (Vpp)"=w319, "ADC Chn. No"=w320, "Sampling Freq String"=w322, "Resolution String"=w323, "Voltage Ref String"=w324) -> ("path to save"=w325:T14, "Save data"=w326:T15)  [unwired: 5 in]
              n81 = Bundle By Name(cluster=T11 {"Fundamental Frequency"=10000.0, "Sampling Frequncy"=250000.0, "No of Harmonics"=9, "Window"=enum."7 Term B-Harris", "Blackman (fundamental power) bins)"=1.0} ("Inputs for Dyanmic para"), "Fundamental Frequency"=w340, "Sampling Frequncy"=w339) -> (w338:T11)
              n82 = call "ADC Data capture and Process Original.vi"("ADC Output Read Method"=T13."Read from Memory", "Select the Tab to project"=T12."SNR", "No.of samples(SNR)"=w337, "Resolution"=w336, "Inputs for Dyanmic para"=w338, "Save data"=w326, "Waveform"=w318, "path to save"=w325) -> ("detected Throughput"=w332:dbl, "Dynamic Parameters"=w335:T16)  [unwired: 13 in, 5 out]
              n83 = Divide(x=w308, y=2.0) -> (x/y=w329:dbl)
              n84 = call "ADC_DynPar_Data_Logging.vi"("Offset (V)"=w329, "detected Throughput"=w332, "Dynamic Parameters"=w335, "error in (no error)"=w333, "Amplitude (Vpp)"=w308, "Ref Voltage"=w331, "Method Cluster In"=w334) -> ("error out"=w327:errorcluster, "End method error"=w328:T1)  [unwired: 3 in]
            }
          }
        }
      }
    }
  }
  "Short Results" <- w3
  "End method error" <- w1
  "error out" <- w2
